vi "rx_ceEq.vi"(5 "symbols":cdb[](array[numeric])) -> (0 "valid?":bool, 1 "neq symbols":cdb[](array[numeric]), 2 "eq symbols":cdb[](array[numeric]))   [LabVIEW 2014]
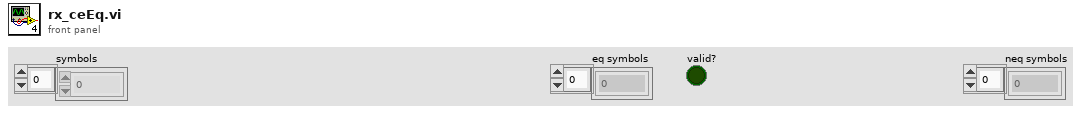
[diagram p1: front panel]
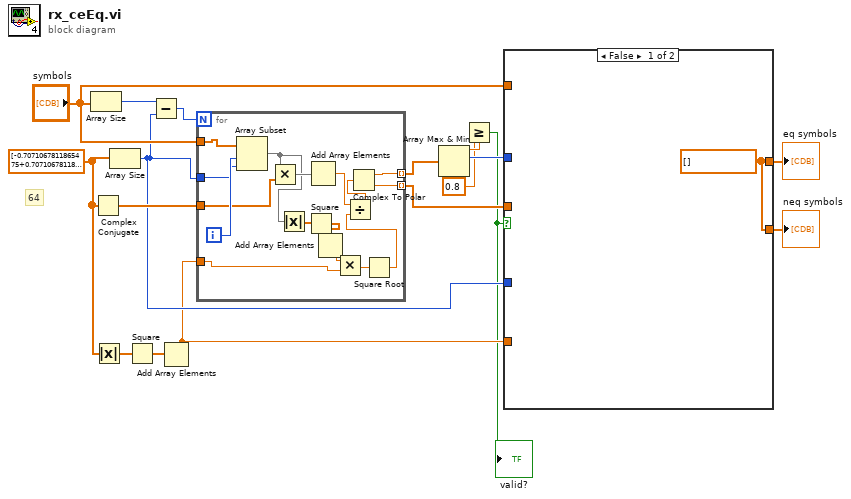
[diagram p0: block diagram]
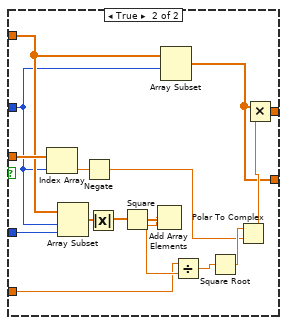
[diagram p2: hidden frame]
diagram:
  w12 = cdb[] [-0.7071067811865475+0.7071067811865476i, 0.7071067811865476+0.7071067811865475i, 0.7071067811865474-0.7071067811865477i, 0.7071067811865476+0.7071067811865475i, -0.7071067811865475+0.7071067811865476i, -0.7071067811865477-0.7071067811865475i, 0.7071067811865476+0.7071067811865475i, -0.7071067811865477-0.7071067811865475i, -0.7071067811865475+0.7071067811865476i, 0.7071067811865476+0.7071067811865475i, 0.7071067811865474-0.7071067811865477i, 0.7071067811865476+0.7071067811865475i, -0.7071067811865475+0.7071067811865476i, -0.7071067811865477-0.7071067811865475i, 0.7071067811865476+0.7071067811865475i, -0.7071067811865477-0.7071067811865475i, -0.7071067811865475+0.7071067811865476i, 0.7071067811865476+0.7071067811865475i, 0.7071067811865474-0.7071067811865477i, 0.7071067811865476+0.7071067811865475i, -0.7071067811865475+0.7071067811865476i, -0.7071067811865477-0.7071067811865475i, 0.7071067811865476+0.7071067811865475i, -0.7071067811865477-0.7071067811865475i, -0.7071067811865475+0.7071067811865476i, 0.7071067811865476+0.7071067811865475i, 0.7071067811865474-0.7071067811865477i, 0.7071067811865476+0.7071067811865475i, -0.7071067811865475+0.7071067811865476i, -0.7071067811865477-0.7071067811865475i, 0.7071067811865476+0.7071067811865475i, -0.7071067811865477-0.7071067811865475i, -0.7071067811865475+0.7071067811865476i, 0.7071067811865476+0.7071067811865475i, 0.7071067811865474-0.7071067811865477i, 0.7071067811865476+0.7071067811865475i, -0.7071067811865475+0.7071067811865476i, -0.7071067811865477-0.7071067811865475i, 0.7071067811865476+0.7071067811865475i, -0.7071067811865477-0.7071067811865475i, -0.7071067811865475+0.7071067811865476i, 0.7071067811865476+0.7071067811865475i, 0.7071067811865474-0.7071067811865477i, 0.7071067811865476+0.7071067811865475i, -0.7071067811865475+0.7071067811865476i, -0.7071067811865477-0.7071067811865475i, 0.7071067811865476+0.7071067811865475i, -0.7071067811865477-0.7071067811865475i, -0.7071067811865475+0.7071067811865476i, 0.7071067811865476+0.7071067811865475i, 0.7071067811865474-0.7071067811865477i, 0.7071067811865476+0.7071067811865475i, -0.7071067811865475+0.7071067811865476i, -0.7071067811865477-0.7071067811865475i, 0.7071067811865476+0.7071067811865475i, -0.7071067811865477-0.7071067811865475i, -0.7071067811865475+0.7071067811865476i, 0.7071067811865476+0.7071067811865475i, 0.7071067811865474-0.7071067811865477i, 0.7071067811865476+0.7071067811865475i, -0.7071067811865475+0.7071067811865476i, -0.7071067811865477-0.7071067811865475i, 0.7071067811865476+0.7071067811865475i, -0.7071067811865477-0.7071067811865475i] ("symbols")
  # "64"
  n1 = Array Size(array="symbols") -> (size(s)=w17:i32)
  n2 = Complex Conjugate(1:w12) -> (0:w15:cdb[])
  n3 = Absolute Value(x=w12) -> (abs(x)=w11:dbl[])
  n4 = Array Size(array=w12) -> (size(s)=w7:i32)
  n5 = Square(x=w11) -> (x^2=w10:dbl[])
  n6 = Subtract(x=w17, y=w7) -> (x-y=w16:i32)
  n7 = Add Array Elements(numeric array=w10) -> (sum=w5:dbl)
  n8 = for {
    N: w16 -> [_]
    tunnel: "symbols" -> [w33]
    tunnel: w15 -> [w30]
    tunnel: w7 -> [w31]
    tunnel: [w28] -> w14 mode=indexing
    tunnel: [w27] -> w13 mode=indexing
    tunnel: w5 -> [w22]
    i -> [w32]
    n9 = Array Subset(array=w33, index=w32, length=w31) -> (w26:cdb[])
    n10 = Multiply(x=w26, y=w30) -> (x*y=w29:cdb[])
    n11 = Absolute Value(x=w26) -> (abs(x)=w25:dbl[])
    n12 = Square(x=w25) -> (x^2=w24:dbl[])
    n13 = Add Array Elements(numeric array=w29) -> (sum=w21:cdb)
    n14 = Add Array Elements(numeric array=w24) -> (sum=w23:dbl)
    n15 = Multiply(x=w23, y=w22) -> (x*y=w20:dbl)
    n16 = Square Root(x=w20) -> (sqrt(x)=w19:dbl)
    n17 = Divide(x=w21, y=w19) -> (x/y=w18:cdb)
    n18 = Complex To Polar(r * e^(i*theta)=w18) -> (r=w28:dbl, theta=w27:dbl)
  }
  n19 = Array Max & Min(array=w14) -> (max value=w4:dbl, max index (indices)=w8:i32)  [unwired: 2 out]
  n20 = Greater Or Equal?(x=w4, y=0.8) -> (x >= y?=w2:bool)
  "valid?" <- w2
  n21 = case shown="False" w2 {
    tunnel: w13 -> [_ w50]
    tunnel: "symbols" -> [_ w48]
    tunnel: w8 -> [_ w47]
    tunnel: w7 -> [_ w46]
    tunnel: [w34 w37] -> w6
    tunnel: w5 -> [_ w36]
    tunnel: [w34 w35] -> w1
    frame False {
      w34 = cdb[] []
    }
    frame True {
      n22 = Index Array(array=w50, index=w47) -> (element=w49:dbl)
      n23 = Array Subset(array=w48, index=w47, length=w46) -> (w45:cdb[])
      n24 = Negate(x=w49) -> (-x=w39:dbl)
      n25 = Absolute Value(x=w45) -> (abs(x)=w44:dbl[])
      n26 = Square(x=w44) -> (x^2=w43:dbl[])
      n27 = Add Array Elements(numeric array=w43) -> (sum=w42:dbl)
      n28 = Array Subset(array=w48, index=w47) -> (w35:cdb[])  [unwired: 1 in]
      n29 = Divide(x=w36, y=w42) -> (x/y=w41:dbl)
      n30 = Square Root(x=w41) -> (sqrt(x)=w40:dbl)
      n31 = Polar To Complex(1:w39, 2:w40) -> (0:w38:cdb)
      n32 = Multiply(x=w35, y=w38) -> (x*y=w37:cdb[])
    }
  }
  "eq symbols" <- w6
  "neq symbols" <- w1
